vi "Angle Vector to Rotation Matrix.vi"(1 "vector":dbl[](array[numeric]), 2 "angle":dbl) -> (0 "rotation matrix":T1)   [LabVIEW 2017, in "NI_Kinematics.lvlib"]
doc: "Returns a <B>rotation matrix</B> that corresponds to a rotation of <B>angle</B> around a <B>vector</B>.\n\n<B>.m file:</B> angvec2r"
uses:
  <vilib>/robotics/Kinematics/NI_Kinematics.lvlib
  <vilib>/Analysis/Matrix/Datatypes/RealMatrix.ctl
  <vilib>/Analysis/_algsub.llb/Real Vector Norm.vi
  <vilib>/Analysis/baseanly.llb/Real Outer Product.vi
  <vilib>/Analysis/Matrix/Numeric/Add/Add - RM,RM.vi
  <vilib>/Analysis/Matrix/Numeric/Multiply/Multiply - R,RM.vi
  <vilib>/Analysis/Matrix/Numeric/Multiply/Multiply - RM,R.vi
  <vilib>/Analysis/7linalg.llb/Create Special Real Matrix.vi
  <vilib>/Analysis/NI_AALBase.lvlib
  <vilib>/Analysis/Matrix/NI_Matrix.lvlib
  <vilib>/Analysis/NI_AALPro.lvlib
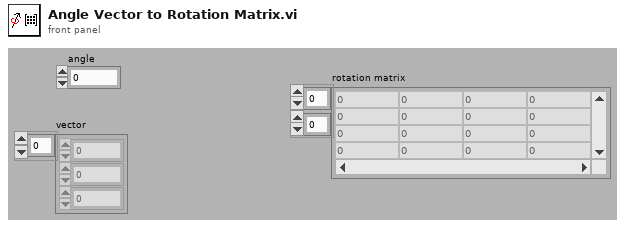
[diagram p1: front panel]
types:
  T1 = typedef "NI_Matrix.lvlib/RealMatrix.ctl" = dbl[][]
  T2 = enum32{"Identity", "Diagonal", "Toepliz", "Vandermonde", "Companion"}
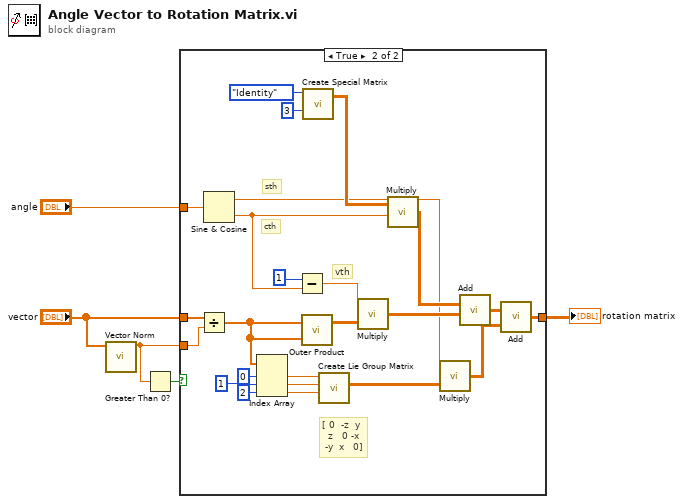
[diagram p0: block diagram]
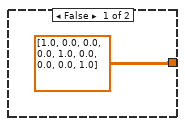
[diagram p2: hidden frame]
diagram:
  n1 = call-poly <vilib>:"Vector Norm.vi"("Input Vector"="vector") -> ("norm"=w1:dbl)  [unwired: 2 in, 8 out]
  n2 = Greater Than 0?(x=w1) -> (x > 0?=w2:bool)
  n3 = case shown="True" w2 {
    tunnel: [dbl[][] [[1.0, 0.0, 0.0], [0.0, 1.0, 0.0], [0.0, 0.0, 1.0]] w21] -> w5
    tunnel: w1 -> [_ w19]
    tunnel: "vector" -> [_ w18]
    tunnel: "angle" -> [_ w15]
    frame False {
    }
    frame True {
      # "vth"
      # "cth"
      # "sth"
      # "[ 0  -z  y\n  z   0 -x\n -y  x   0]"
      n4 = Divide(x=w18, y=w19) -> (x/y=w11:dbl[])
      n5 = Sine & Cosine(0:w15) -> (1:w16:dbl, 2:w17:dbl)
      n6 = Index Array(array=w11, index #1=0 ("index"), index #2=1 ("index"), index #3=2 ("index")) -> (element #1=w10:dbl, element #2=w9:dbl, element #3=w8:dbl)
      n7 = Subtract(x=1, y=w17) -> (x-y=w29:dbl)
      n8 = call-poly <vilib>:"Outer Product.vi"("Y Vector"=w11, "X Vector"=w11) -> ("Outer Product"=w25:T1)  [unwired: 1 out]
      n9 = call-poly <vilib>:"Create Special Matrix.vi"("matrix type"=T2."Identity", "matrix size"=3) -> ("Special Matrix"=w26:T1)  [unwired: 2 in, 2 out]
      n10 = call <vilib>:"Create Lie Group Matrix.vi"("z"=w8, "y"=w9, "x"=w10) -> ("real matrix"=w7:T1)  [unwired: 8 in]
      n11 = call-poly <vilib>:"Multiply.vi"("Real Matrix A"=w25, "Real Scalar c"=w29) -> ("c * A"=w23:T1)
      n12 = call-poly <vilib>:"Multiply.vi"("Real Scalar c"=w17, "Real Matrix A"=w26) -> ("A * c"=w24:T1)
      n13 = call-poly <vilib>:"Multiply.vi"("Real Matrix A"=w7, "Real Scalar c"=w16) -> ("c * A"=w20:T1)
      n14 = call-poly <vilib>:"Add.vi"("Real Matrix B"=w23, "Real Matrix A"=w24) -> ("A + B"=w22:T1)
      n15 = call-poly <vilib>:"Add.vi"("Real Matrix B"=w20, "Real Matrix A"=w22) -> ("A + B"=w21:T1)
    }
  }
  "rotation matrix" <- w5
